vi "Functional Test Info Dialog.vi"(5 "Functional Test Data In":T1) -> (4 "Type Name Out":string, 6 "Functional Test Data":T1, 8 "Cancelled?":bool)   [LabVIEW 2019]
uses:
  Type Defs and Controls/Functional Info.ctl
panel:
  in  "Temperature":dbl step=0.1 format="%.1f Deg C"
  in  "Voltage":dbl min=0.0 step=0.01 format="%.1f V"
  in  "Technician Name":string
  in  "Cancel":bool
  in  "OK":bool
  # "Please Enter Test Information:"
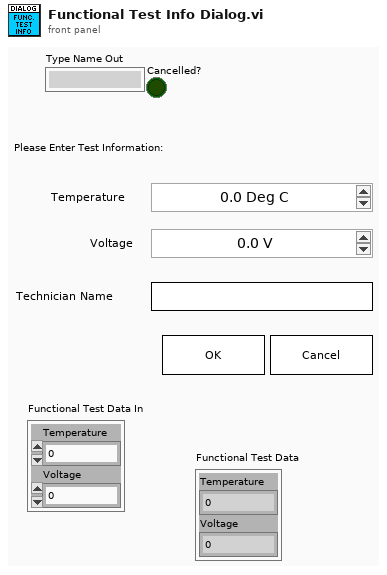
[diagram p1: front panel]
types:
  T1 = typedef "Functional Info.ctl" = cluster{"Temperature":dbl, "Voltage":dbl}
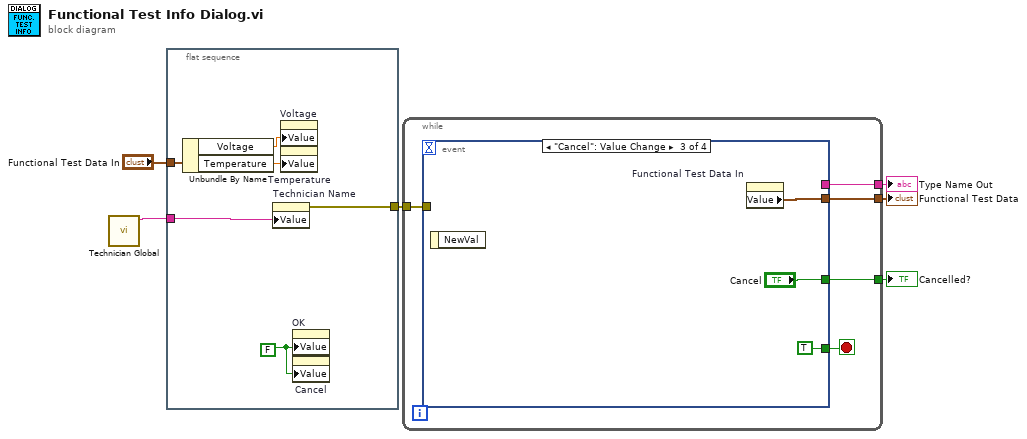
[diagram p0: block diagram]
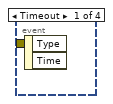
[diagram p2: hidden frame]
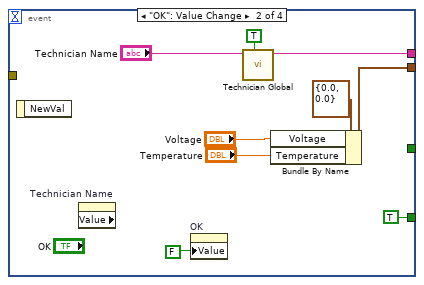
[diagram p3: hidden frame]
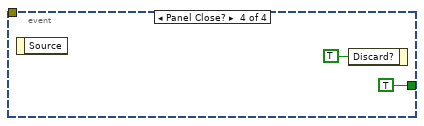
[diagram p4: hidden frame]
diagram:
  n1 = call "Technician Global.vi"() -> ("Technician Name"=w3:string)  [unwired: 11 in]
  n2 = flat-sequence {
    tunnel: [w12] -> w4
    tunnel: w3 -> [w10]
    tunnel: "Functional Test Data In" -> [w9]
    frame #0 {
      w11 = FALSE ("Key Focus")
      n3 = Unbundle By Name(w9) -> ("Voltage"=w7:dbl, "Temperature"=w8:dbl)
      n4 = property on="Technician Name" class="Str"("Value"=w10) -> (error out=w12:errorcluster)  [unwired: 2 in, 1 out]
      n5 = property on="Voltage" class="DigNum (strict)"("Value"=w7) -> ()  [unwired: 2 in, 2 out]
      n6 = property on="Temperature" class="DigNum (strict)"("Value"=w8) -> ()  [unwired: 2 in, 2 out]
      n7 = property on="OK" class="Bool (strict)"("Value"=w11) -> ()  [unwired: 2 in, 2 out]
      n8 = property on="Cancel" class="Bool (strict)"("Value"=w11) -> ()  [unwired: 2 in, 2 out]
    }
  }
  n9 = while {
    tunnel: [w17] -> w6
    tunnel: [w16] -> w5
    tunnel: w4 -> [w15]
    tunnel: [w13] -> w2
    stop <- w14 stop-if-true
    n10 = event shown="[2] \"Cancel\": Value Change" {
      selector: _ -> [_ _ _ _]
      dyn-events: _ -> [_ _ _ _]
      timeout: _ -> [_ _ _ _]
      tunnel: [_ _ "Cancel" TRUE ("Cancel")] -> w17
      tunnel: [_ w22 _ _] -> w16
      tunnel: w15 -> [_ _ _ _]
      tunnel: [_ TRUE TRUE _] -> w14
      tunnel: [_ w18 w27 _] -> w13
      event Timeout {
        n11 = event-data() -> ()  [unwired: 1 in, 2 out]
      }
      event "OK": Value Change {
        n12 = event-data() -> ()  [unwired: 1 in, 1 out]
        n13 = property on="Technician Name" class="Str" props=["Value"]() -> ()  [unwired: 2 in, 3 out]
        n14 = property on="OK" class="Bool (strict)"("Value"=FALSE ("Key Focus")) -> ()  [unwired: 2 in, 2 out]
        n15 = call "Technician Global.vi"("Write? (F)"=TRUE, "Technician Name"="Technician Name") -> ("Technician Name"=w22:string)  [unwired: 9 in]
        n16 = Bundle By Name(cluster=T1 {"Temperature"=0.0, "Voltage"=0.0} ("Functional Test Data"), "Voltage"="Voltage", "Temperature"="Temperature") -> (w18:T1)
      }
      event "Cancel": Value Change {
        n17 = event-data() -> ()  [unwired: 1 in, 1 out]
        n18 = property on="Functional Test Data In" class="Clust (strict)"() -> ("Value"=w27:T1)  [unwired: 2 in, 2 out]
      }
      event Panel Close? {
        n19 = event-data() -> ()  [unwired: 1 in, 1 out]
        n20 = event-data("Discard?"=TRUE) -> ()  [unwired: 1 in, 1 out]
      }
    }
  }
  "Cancelled?" <- w6
  "Type Name Out" <- w5
  "Functional Test Data" <- w2
